vi "Config CDMA2000 Spreading.vi"(0 "VISA Resource Name":refnum<visa-resource-name>, 5 "Type  (0:Direct)":enum16{"Direct", "Multi Carrier"}(ring), 7 "Rate (1)":i32=1, 9 "MCarrier Spaccing  (0: 1.23 MHz)":enum16{"1.23 MHz", "1.25 MHz"}(ring), 11 "error in (no error)":errorcluster {"code" format="%.0x"}) -> (4 "VISA Resource Name Out":refnum<visa-resource-name>, 15 "error out":errorcluster {"code" format="%.0x"})   [LabVIEW 2012, in "Agilent ESG Series.lvlib"]
doc: "This VI configures CDMA2000 spreading parameters.\n\nNotes:\n(1) This VI is supported for Agilent E44xxB with option 101 or E4438C with option 401 only."
uses:
  <instrlib>/Agilent ESG Series/Agilent ESG Series.lvlib
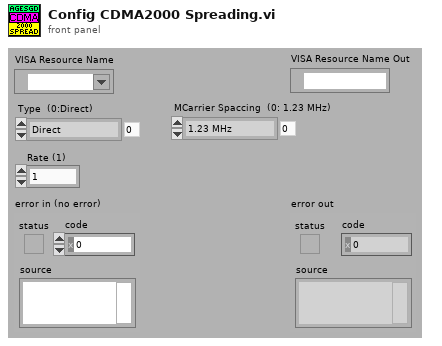
[diagram p1: front panel]
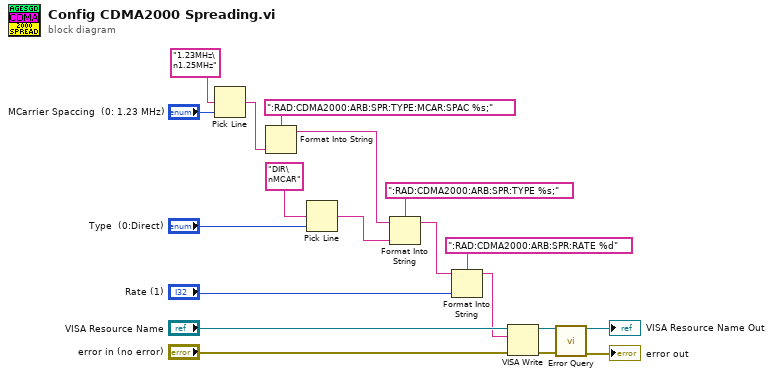
[diagram p0: block diagram]
diagram:
  n1 = Pick Line(multi-line string="1.23MHz\n1.25MHz", line index="MCarrier Spaccing  (0: 1.23 MHz)") -> (output string=w11:string)  [unwired: 1 in]
  n2 = Format Into String(format string=":RAD:CDMA2000:ARB:SPR:TYPE:MCAR:SPAC %s;", w11) -> (resulting string=w1:string)  [unwired: 2 in, 1 out]
  n3 = Pick Line(multi-line string="DIR\nMCAR", line index="Type  (0:Direct)") -> (output string=w5:string)  [unwired: 1 in]
  n4 = Format Into String(format string=":RAD:CDMA2000:ARB:SPR:TYPE %s;", initial string=w1, w5) -> (resulting string=w2:string)  [unwired: 1 in, 1 out]
  n5 = Format Into String(format string=":RAD:CDMA2000:ARB:SPR:RATE %d", initial string=w2, "Rate (1)") -> (resulting string=w3:string)  [unwired: 1 in, 1 out]
  n6 = VISA Write(VISA resource name="VISA Resource Name", write buffer=w3, error in (no error)="error in (no error)") -> (VISA resource name out=w15:refnum<visa-resource-name>, error out=w14:errorcluster)  [unwired: 1 out]
  n7 = call <instrlib>:"Error Query.vi"("VISA Resource Name"=w15, "error in (no error)"=w14) -> ("VISA Resource Name Out"=→"VISA Resource Name Out":refnum<visa-resource-name>, "error out"=→"error out":errorcluster)  [unwired: 10 in, 2 out]
